vi "SwerveMath.vi"(0 "X-Axis":dbl, 2 "Y-Axis":dbl, 4 "Turn":dbl, 6 "CentricToggle":bool) -> (20 "FrontLeftAngle":dbl, 21 "FrontLeftDrive":dbl, 22 "FrontRightAngle":dbl, 23 "FrontRightDrive":dbl, 24 "RearLeftAngle":dbl, 25 "RearLeftDrive":dbl, 26 "RearRightAngle":dbl, 27 "RearRightDrive":dbl)   [LabVIEW 2018]
uses:
  <vilib>/Rock Robotics/Network Tables/NT Read Boolean.vi
  Robot Global Data.vi
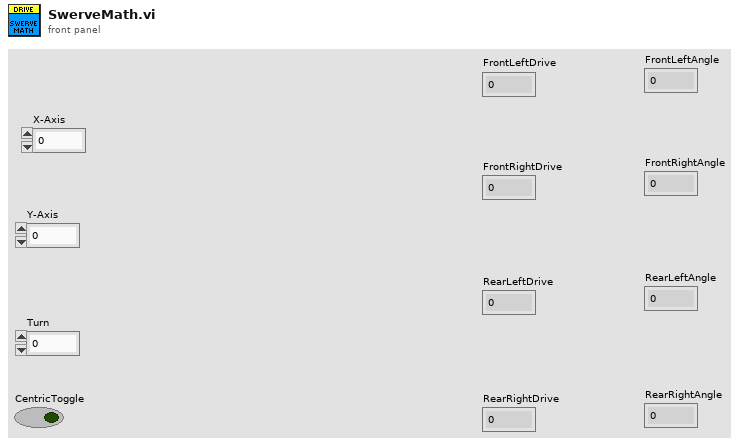
[diagram p1: front panel]
types:
  T1 = typedef "WPI_DriverStationRobotMode2.ctl" = enum16{"Autonomous Disabled", "Autonomous Enabled", "Teleop Disabled", "Teleop Enabled", "Disconnected", "Finish", "Test Disabled", "Test Enabled", "Emergency Stopped"}
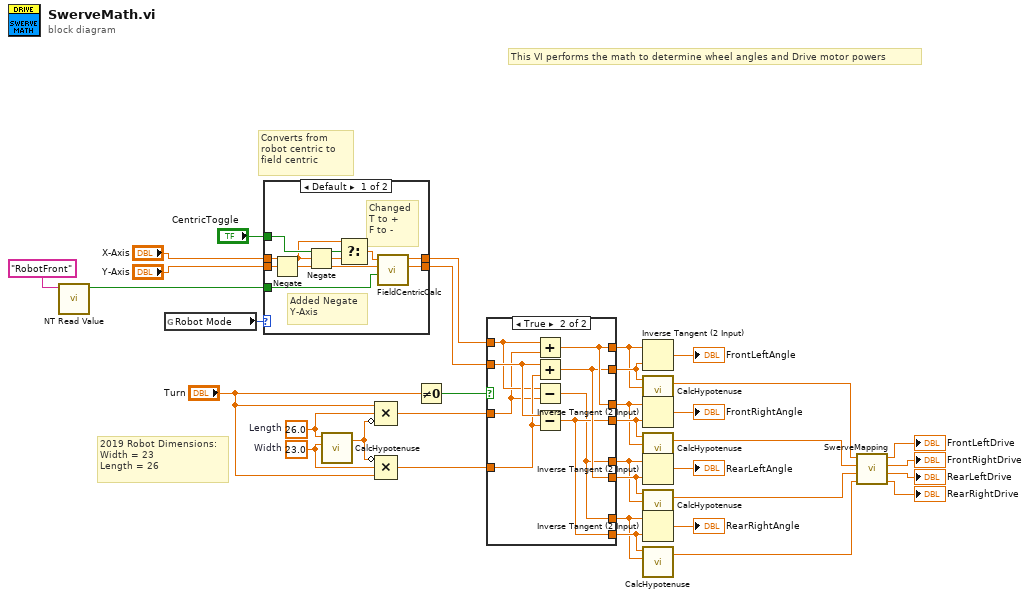
[diagram p0: block diagram]
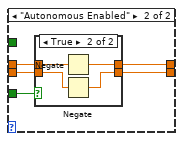
[diagram p2: hidden frame]
diagram:
  w31 = 26.0  # Length
  w30 = 23.0  # Width
  # "2019 Robot Dimensions:\nWidth = 23\nLength = 26"
  # "This VI performs the math to determine wheel angles and Drive motor powers"
  # "Converts from robot centric to field centric"
  n1 = call-poly <vilib>:"NT Read Value.vi"("Name"="RobotFront") -> ("Boolean"=w2:bool)  [unwired: 9 in, 1 out]
  n2 = global read "Robot Global Data.vi" "Robot Mode"() -> (w4:T1)
  n3 = case shown="Default" w4 {
    tunnel: "Y-Axis" -> [w37 w45]
    tunnel: "X-Axis" -> [w38 w47]
    tunnel: [w44 w48] -> w26
    tunnel: [w43 w46] -> w25
    tunnel: w2 -> [w42 w49]
    tunnel: "CentricToggle" -> [w41 _]
    frame Default {
      # "Added Negate\nY-Axis"
      # "Changed\nT to +\nF to -"
      n4 = Negate(x=w37) -> (-x=w36:dbl)
      n5 = Negate(x=w38) -> (-x=w39:dbl)
      n6 = Select(t=w38, s=w41, f=w39) -> (s? t:f=w40:dbl)
      n7 = call "FieldCentricCalc.vi"("RobotFront"=w42, "y_in"=w36, "x_in"=w40) -> ("y_out"=w43:dbl, "x_out"=w44:dbl)  [unwired: 7 in]
    }
    frame "Autonomous Enabled" {
      n8 = case shown="True" w49 {
        tunnel: [w51 w55] -> w48
        tunnel: w47 -> [w51 w54]
        tunnel: [w50 w53] -> w46
        tunnel: w45 -> [w50 w52]
        frame False {
        }
        frame True {
          n9 = Negate(x=w54) -> (-x=w55:dbl)
          n10 = Negate(x=w52) -> (-x=w53:dbl)
        }
      }
    }
  }
  n11 = call "CalcHypotenuse.vi"("b"=w30, "a"=w31) -> ("hypotenuse"=w32:dbl)  [unwired: 3 in]
  n12 = Compound Arithmetic op=MULTIPLY("Turn", w31, invert w32) -> (w27:dbl)
  n13 = Compound Arithmetic op=MULTIPLY(invert w32, w30, "Turn") -> (w28:dbl)
  n14 = Not Equal To 0?(x="Turn") -> (x != 0?=w33:bool)
  n15 = case shown="True" w33 {
    tunnel: w25 -> [w56 w65]
    tunnel: w28 -> [_ w64]
    tunnel: w26 -> [w57 w63]
    tunnel: [w57 w61] -> w23
    tunnel: [w56 w60] -> w24
    tunnel: [w57 w61] -> w21
    tunnel: [w56 w59] -> w22
    tunnel: [w57 w58] -> w19
    tunnel: [w56 w60] -> w20
    tunnel: [w57 w58] -> w17
    tunnel: [w56 w59] -> w18
    tunnel: w27 -> [_ w62]
    frame False {
    }
    frame True {
      n16 = Add(x=w63, y=w62) -> (x+y=w61:dbl)
      n17 = Add(x=w65, y=w64) -> (x+y=w60:dbl)
      n18 = Subtract(x=w63, y=w62) -> (x-y=w58:dbl)
      n19 = Subtract(x=w65, y=w64) -> (x-y=w59:dbl)
    }
  }
  n20 = Inverse Tangent (2 Input)(1:w24, 2:w23) -> (0:→"FrontLeftAngle":dbl)
  n21 = call "CalcHypotenuse.vi"("b"=w23, "a"=w24) -> ("hypotenuse"=w12:dbl)  [unwired: 3 in]
  n22 = Inverse Tangent (2 Input)(1:w22, 2:w21) -> (0:→"FrontRightAngle":dbl)
  n23 = call "CalcHypotenuse.vi"("b"=w21, "a"=w22) -> ("hypotenuse"=w11:dbl)  [unwired: 3 in]
  n24 = Inverse Tangent (2 Input)(1:w20, 2:w19) -> (0:→"RearLeftAngle":dbl)
  n25 = call "CalcHypotenuse.vi"("b"=w19, "a"=w20) -> ("hypotenuse"=w10:dbl)  [unwired: 3 in]
  n26 = Inverse Tangent (2 Input)(1:w18, 2:w17) -> (0:→"RearRightAngle":dbl)
  n27 = call "CalcHypotenuse.vi"("b"=w17, "a"=w18) -> ("hypotenuse"=w9:dbl)  [unwired: 3 in]
  n28 = call "SwerveMapping.vi"("RearRightDriveIn"=w9, "RearLeftDriveIn"=w10, "FrontRightDriveIn"=w11, "FrontLeftDriveIn"=w12) -> ("RearRightDriveOut"=→"RearRightDrive":dbl, "RearLeftDriveOut"=→"RearLeftDrive":dbl, "FrontRightDriveOut"=→"FrontRightDrive":dbl, "FrontLeftDriveOut"=→"FrontLeftDrive":dbl)  [unwired: 4 in]
